vi "HTS_FULL_PLATE_CONSTANT.vi"() -> (0 "Array":T1[](array[typedef]))   [LabVIEW 2009]
uses:
  HTS_WELL.ctl
  HTS_COLUMN.ctl
  HTS_ROW.ctl
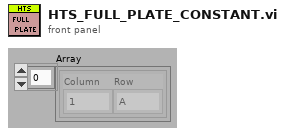
[diagram p1: front panel]
types:
  T1 = typedef "HTS_WELL.ctl" = cluster{"Column":T2, "Row":T3}
  T2 = typedef "HTS_COLUMN.ctl" = enum16{"1", "2", "3", "4", "5", "6", "7", "8", "9", "10", "11", "12"}
  T3 = typedef "HTS_ROW.ctl" = enum16{"A", "B", "C", "D", "E", "F", "G", "H"}
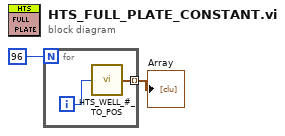
[diagram p0: block diagram]
diagram:
  n1 = for {
    N: 96 -> [_]
    tunnel: [w3] -> w1 mode=indexing
    i -> [w4]
    n2 = call "HTS_WELL_#_TO_POS.vi"("Well Number (0-95)"=w4) -> ("Well Position"=w3:T1)  [unwired: 4 out]
  }
  "Array" <- w1
